vi "FFT FPGA Initialize.vi"(8 "error in (no error)":errorcluster, 11 "Refnum in":refnum<k20>) -> (0 "error out":errorcluster, 3 "Refnum out":refnum<k20>)   [LabVIEW 2019]
uses:
  <vilib>/rvi/interface/common/niFpgaWaitOnOcc.vi
  <vilib>/Utility/error.llb/Error Cluster From Error Code.vi
  <vilib>/FPGAPlugInAG/Dynamic/niLvFpga_Run_Dynamic.vi
  <vilib>/rvi/interface/nirviMethod/nirviMethod.xnode
  <vilib>/FPGAPlugInAG/Dynamic/niLvFpga_StartFifo_Dynamic.vi
  <vilib>/rvi/errors/niLvFpgaMergeErrorWithErrorCode.vi
  <vilib>/FPGAPlugInAG/Dynamic/niLvFpga_ConfigureFifo_Dynamic.vi
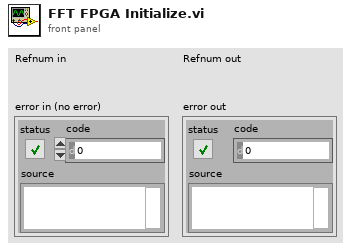
[diagram p1: front panel]
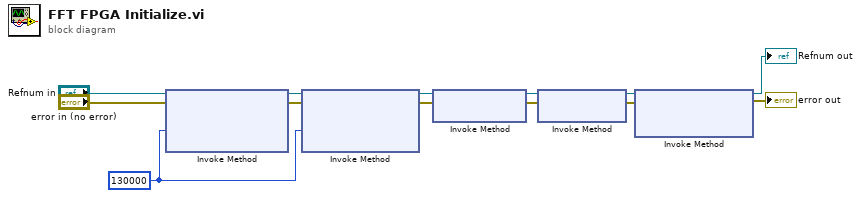
[diagram p0: block diagram]
diagram:
  w3 = u32 130000
  n1 = xnode "Invoke Method"("FPGA VI Reference In"="Refnum in", "error in"="error in (no error)", "Requested Depth"=w3) -> ("FPGA VI Reference Out"=w7:refnum<k20>, "error out"=w5:errorcluster)  [unwired: 1 out]
  n2 = xnode "Invoke Method"("FPGA VI Reference In"=w7, "error in"=w5, "Requested Depth"=w3) -> ("FPGA VI Reference Out"=w6:refnum<k20>, "error out"=w4:errorcluster)  [unwired: 1 out]
  n3 = xnode "Invoke Method"("FPGA VI Reference In"=w6, "error in"=w4) -> ("FPGA VI Reference Out"=w10:refnum<k20>, "error out"=w8:errorcluster)
  n4 = xnode "Invoke Method"("FPGA VI Reference In"=w10, "error in"=w8) -> ("FPGA VI Reference Out"=w11:refnum<k20>, "error out"=w9:errorcluster)
  n5 = xnode "Invoke Method"("FPGA VI Reference In"=w11, "error in"=w9) -> ("FPGA VI Reference Out"=→"Refnum out":refnum<k20>, "error out"=→"error out":errorcluster)  [unwired: 1 in]
